vi "RP Read Temperature TCP.vi"(8 "Error In":errorcluster, 9 "timeout ms (25000)":i32, 11 "connection ID":refnum<k5>) -> (0 "error out":errorcluster, 2 "Thermometer":dbl(slide)=48.847186279148 scale=0.0..100.0, 3 "connection ID out":refnum<k5>)   [LabVIEW 2019]
uses:
  RP Command.ctl
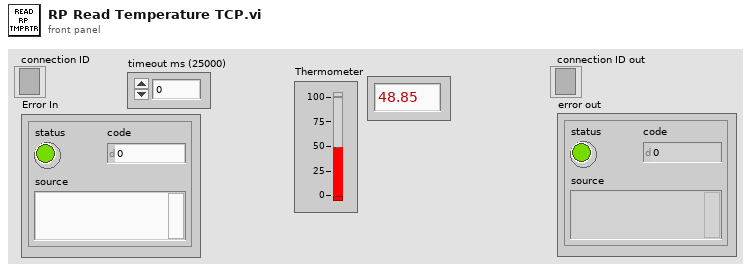
[diagram p1: front panel]
types:
  T1 = enum16{"big-endian, network order", "native, host order", "little-endian"}
  T2 = typedef "RP Command.ctl" = enum16{"Reset", "Read IDN", "Stop server", "Get status", "Get temperature", "Connect client", "Arm", "Software trigger", "Get whole buffer", "Get chunk", "System call", "Get config", "Set config", "Recieve data", "Recieve Calibartion", "Transmit data"}
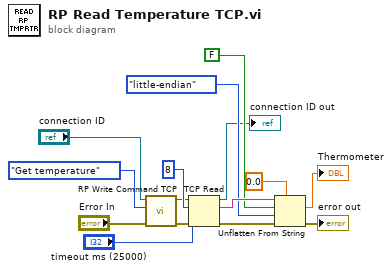
[diagram p0: block diagram]
diagram:
  n1 = call "RP Write Command TCP.vi"("Error In"="Error In", "Command number"=RP_Command."Get temperature", "connection ID"="connection ID") -> ("Error Out"=w8:errorcluster, "connection ID out"=w7:refnum<k5>)  [unwired: 6 in, 1 out]
  n2 = TCP Read(connection ID=w7, bytes to read=8, error in (no error)=w8, 9:"timeout ms (25000)") -> (connection ID out=→"connection ID out":refnum<k5>, data out=w14:string, error out=w12:errorcluster)  [unwired: 1 in]
  n3 = Unflatten From String(type=0.0, binary string=w14, data includes array or string size? (T)=FALSE, byte order (0:big-endian, network order)=T1."little-endian", error in (no error)=w12) -> (value=→"Thermometer":dbl, error out=→"error out":errorcluster)  [unwired: 1 out]
